vi "SetParam.vi"(8 "error in (no error)":errorcluster caption="entrée d'erreur (pas d'erreur)", 10 "sigmoid_kernel":cluster{"gamma":string, "coef0":dbl}={"gamma"="None", "coef0"=1.0}, 11 "Sigmoid_kernel.lvclass":refnum<class "Sigmoid_kernel.lvclass">) -> (0 "error out":errorcluster caption="sortie d'erreur", 3 "Sigmoid_kernel.lvclass":refnum<class "Sigmoid_kernel.lvclass">)   [LabVIEW 2020, in "Sigmoid_kernel.lvclass"]
doc: "Set Parameters"
uses:
  Sigmoid_kernel.lvclass
  Sigmoid_kernel.lvclass/Sigmoid_kernel.ctl
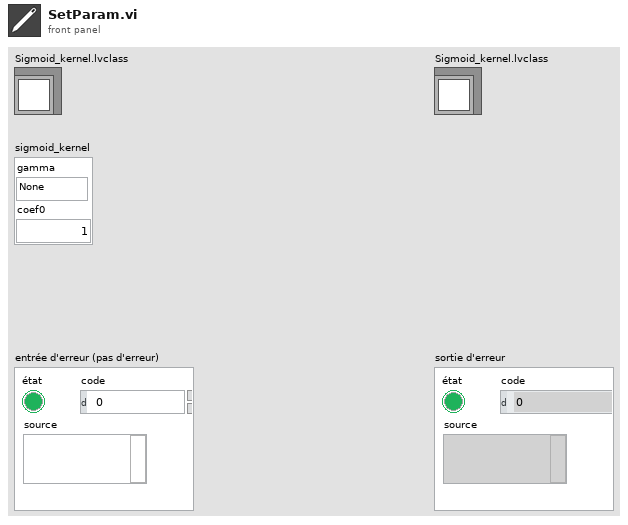
[diagram p1: front panel]
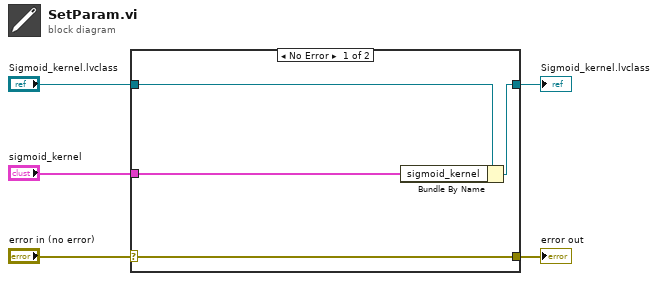
[diagram p0: block diagram]
diagram:
  n1 = case shown="No Error" "error in (no error)" {
    selector: "error in (no error)" -> [w9 w10]
    tunnel: [w9 w10] -> w4
    tunnel: [w7 w11] -> w2
    tunnel: "Sigmoid_kernel.lvclass" -> [w8 w11]
    tunnel: "sigmoid_kernel" -> [w6 _]
    frame No Error {
      n2 = Bundle By Name(cluster=w8, "sigmoid_kernel"=w6) -> (w7:refnum<class "Sigmoid_kernel.lvclass">)
    }
    frame Error {
    }
  }
  "error out" <- w4
  "Sigmoid_kernel.lvclass" <- w2
